vi "GetHelp.vi"(11 "UniquifyFullyQualifiedVIName in":refnum<class "UniquifyFullyQualifiedVIName.lvclass">) -> (2 "Help":string, 3 "UniquifyFullyQualifiedVIName out":refnum<class "UniquifyFullyQualifiedVIName.lvclass">)   [LabVIEW 2015, in "UniquifyFullyQualifiedVIName.lvclass"]
uses:
  UniquifyFullyQualifiedVIName.lvclass
  <nishared>/LabVIEW CLI/Operations/CoreOperation/CoreOperation.lvclass
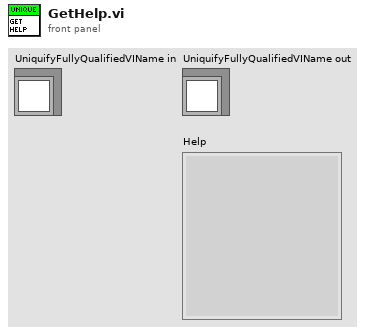
[diagram p1: front panel]
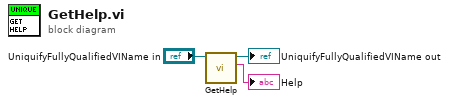
[diagram p0: block diagram]
diagram:
  n1 = call-parent "GetHelp.vi"("CoreOperation in"="UniquifyFullyQualifiedVIName in") -> ("Help"=→"Help":string, "CoreOperation out"=→"UniquifyFullyQualifiedVIName out":refnum<class "UniquifyFullyQualifiedVIName.lvclass">)  [unwired: 9 in]
